vi "Main.vi"() -> ()   [LabVIEW 2013]
panel:
  in  "stop":bool
  out "Status:":string
  out "User Path Input":string
  out "Path":path
  in  "Notes":string
  out "Progress (At This Temp)":u8(slide) scale=0.0..100.0
  out "Progress (Total)":u8(slide) scale=0.0..100.0
  out "RTD Index":i32
  out "Relay Index":i32
  out "temp index":i32
  in  "Wirings":string[](array[string])=["2 Wire", "3 Wire"]
  in  "Loads":dbl[](array[numeric])=[0.0, 300.0]
  in  "Samples per Reading":dbl=1000.0
  in  "Soak Temps":dbl[](array[numeric])=[25.0, 35.0]
  in  "Multimeter USB Port":refnum<visa-resource-name>="USB0::0x0957::0x0607::MY47028683::INSTR"
  in  "Settling Time (s)":dbl=10.0
  in  "Relay Box COM Port":refnum<visa-resource-name>="COM4"
  in  "Relay Settings":u8[](array[numeric])=[0, 2, 8, 10] format="%08b"
  in  "Burster COM Port":refnum<visa-resource-name>="COM6"
  in  "Power Supply COM Port":refnum<visa-resource-name>="COM8"
  in  "RTD Temps":dbl[](array[numeric])=[50.0, 60.0, 70.0, 80.0, 90.0, 100.0, 110.0]
  in  "Voltages":dbl[](array[numeric])=[18.0, 24.0, 36.0]
  in  "Thermal Soak Time (m)":dbl=1.0
  in  "Thermal Chamber COM Port":refnum<visa-resource-name>="COM7"
  # "IFM TEMPERATURE SENSOR TEST PLATFORM"
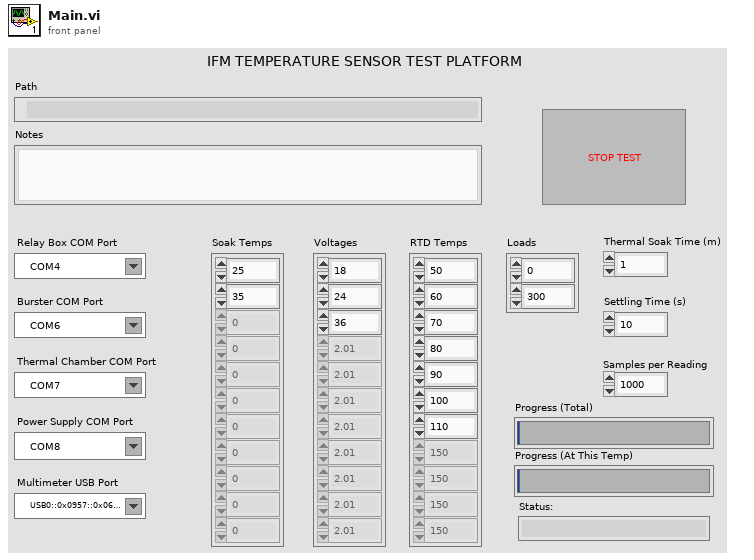
[diagram p1: front panel]
types:
  T1 = enum16{"Left Button", "Center Button", "Right Button", "Window Close"}
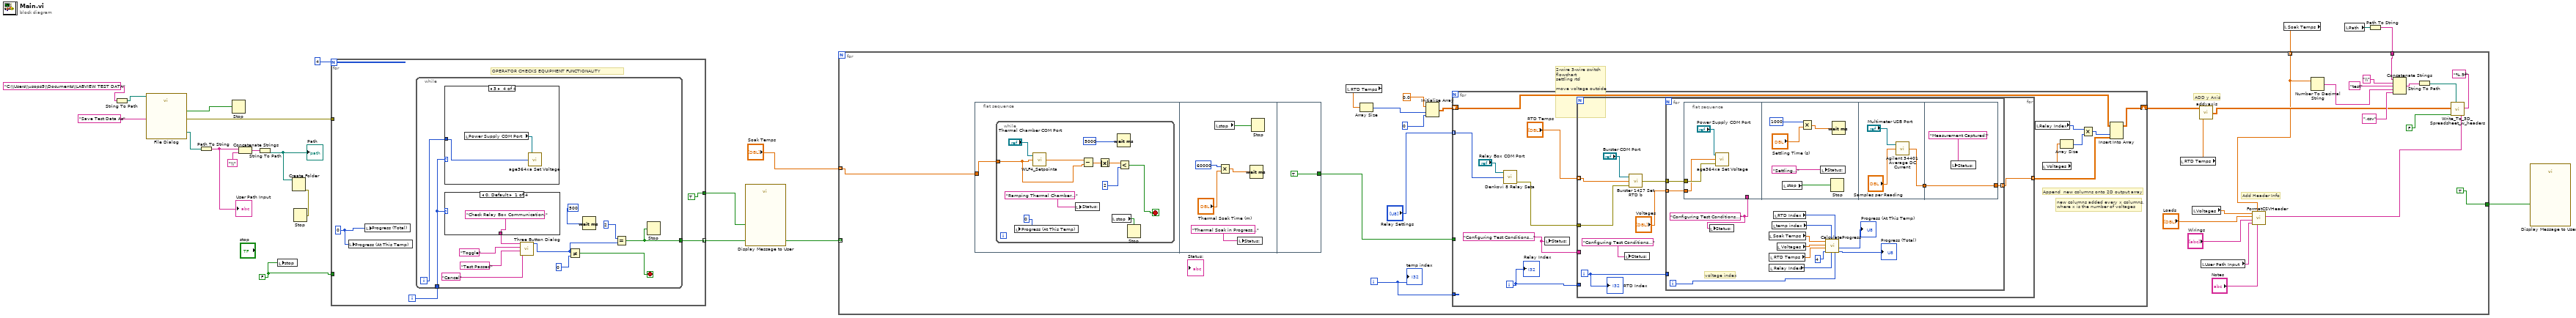
[diagram p0: block diagram]
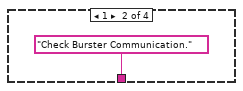
[diagram p2: hidden frame]
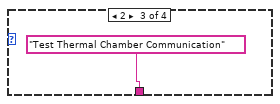
[diagram p3: hidden frame]
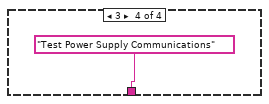
[diagram p4: hidden frame]
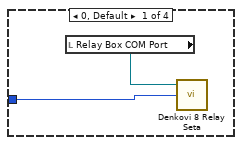
[diagram p5: hidden frame]
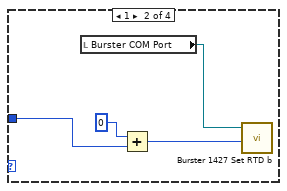
[diagram p6: hidden frame]
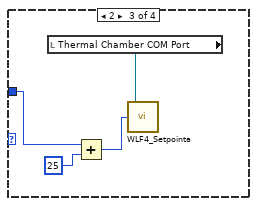
[diagram p7: hidden frame]
diagram:
  w2 = FALSE
  n1 = String To Path(string="C:\\Users\\usops5\\Documents\\LABVIEW TEST DATA") -> (path=w11:path)
  n2 = call "File Dialog"("start path"=w11, "prompt"="Save Test Data As") -> ("selected path"=w13:path, "cancelled"=w14:bool, "error out"=w15:errorcluster)  [unwired: 10 in, 1 out]
  n3 = Path To String(path=w13) -> (string=w4:string)
  "User Path Input" <- w4
  n4 = Stop(stop? (T)=w14) -> ()
  n5 = Concatenate Strings(w4, "\\") -> (w10:string)
  n6 = String To Path(string=w10) -> (path=w7:path)
  "Path" <- w7
  n7 = local write "stop"(w2) -> ()
  n8 = Create Folder(path (use dialog)=w7) -> (error out=w6:errorcluster)  [unwired: 2 in, 2 out]
  n9 = Stop(stop? (T)=w6) -> ()
  n10 = for {
    N: 4 -> [_]
    tunnel: [w23] -> w17 mode=indexing
    tunnel: w15 -> [_]
    tunnel: [TRUE] -> w3
    tunnel: w2 -> [_]
    i -> [w24]
    w21 = 0
    # "OPERATOR CHECKS EQUIPMENT FUNCTIONALITY"
    n11 = local write "Progress (At This Temp)"(w21) -> ()
    n12 = local write "Progress (Total)"(w21) -> ()
    n13 = while {
      tunnel: w24 -> [w26]
      tunnel: [w27] -> w23
      i -> [w30]
      stop <- w32 stop-if-true
      n14 = case shown="3" w26 {
        tunnel: w30 -> [w41 w46 w50 w52]
        frame 0, Default {
          n15 = local read "Relay Box COM Port"() -> (w42:refnum<visa-resource-name>)
          n16 = call "Denkovi 8 Relay Seta.vi"("Numeric"=w41, "VISA resource name"=w42) -> ()  [unwired: 3 in, 1 out]
        }
        frame 1 {
          n17 = local read "Burster COM Port"() -> (w43:refnum<visa-resource-name>)
          n18 = Add(x=0, y=w46) -> (x+y=w44:i32)
          n19 = call "Burster 1427 Set RTD b.vi"("RTD Setting"=w44, "VISA resource name"=w43) -> ()  [unwired: 1 in, 1 out]
        }
        frame 2 {
          n20 = local read "Thermal Chamber COM Port"() -> (w47:refnum<visa-resource-name>)
          n21 = Add(x=w50, y=25) -> (x+y=w48:i32)
          n22 = call "WLF4_Setpointa.vi"("Set Point 1"=w48, "Instrument Resource Name"=w47) -> ()  [unwired: 3 in, 1 out]
        }
        frame 3 {
          n23 = local read "Power Supply COM Port"() -> (w51:refnum<visa-resource-name>)
          n24 = call "age364xa Set Voltage.vi"("Voltage level (0.0 Volts)"=w52, "Instrument Resource Name (\"GPIB::5::INSTR\")"=w51) -> ()  [unwired: 1 in, 1 out]
        }
      }
      n25 = case shown="0, Default" w26 {
        tunnel: ["Check Relay Box Communication." "Check Burster Communication." "Test Thermal Chamber Communication" "Test Power Supply Communications"] -> w25
        frame 0, Default {
        }
        frame 1 {
        }
        frame 2 {
        }
        frame 3 {
        }
      }
      n26 = call <vilib>:"Three Button Dialog.vi"("Right Button Text (\"Cancel\")"="Cancel", "Center Button Text (\"No\")"="Test Passed", "Left Button Text (\"Yes\")"="Toggle", "message"=w25) -> ("Which Button?"=w28:T1)  [unwired: 7 in]
      n27 = Not Equal?(x=w28, y=0) -> (x != y?=w32:bool)
      n28 = Wait (ms)(milliseconds to wait=500) -> ()  [unwired: 1 out]
      n29 = Equal?(x=2, y=w28) -> (x = y?=w27:bool)
      n30 = Stop(stop? (T)=w27) -> ()
    }
  }
  n31 = call "Display Message to User"("Enable"=w3) -> ()  [unwired: 9 in, 2 out]
  n32 = local read "Soak Temps"() -> (w20:dbl[])
  n33 = local read "Path"() -> (w8:path)
  n34 = Path To String(path=w8) -> (string=w5:string)
  n35 = for {
    tunnel: "Soak Temps" -> [w81] mode=indexing
    tunnel: w5 -> [w54]
    tunnel: w20 -> [w69] mode=indexing
    tunnel: w17 -> [_] mode=indexing
    tunnel: [TRUE] -> w1
    i -> [w56]
    # "2-wire 3-wire switch\nflowchart\nsettling rtd\n\nmove voltage outside"
    # "ADD y Axis"
    # "Add Header Info"
    n36 = flat-sequence {
      tunnel: w81 -> [w82]
      tunnel: [TRUE] -> w59
      frame #0 {
        n37 = while {
          tunnel: w82 -> [w86]
          stop <- w89 stop-if-true
          n38 = local write "Progress (At This Temp)"(0) -> ()
          n39 = call "WLF4_Setpointa.vi"("Set Point 1"=w86, "Instrument Resource Name"="Thermal Chamber COM Port") -> ("Measured Temp"=w93:dbl)  [unwired: 3 in]
          n40 = local write "Status:"("Ramping Thermal Chamber...") -> ()
          n41 = Subtract(x=w93, y=w86) -> (x-y=w92:dbl)
          n42 = Absolute Value(x=w92) -> (abs(x)=w91:dbl)
          n43 = local read "stop"() -> (w83:bool)
          n44 = Wait (ms)(milliseconds to wait=5000) -> ()  [unwired: 1 out]
          n45 = Less?(x=w91, y=2) -> (x < y?=w89:bool)
          n46 = Stop(stop? (T)=w83) -> ()
        }
      }
      frame #1 {
        n47 = local read "stop"() -> (w94:bool)
        n48 = Multiply(x=60000, y="Thermal Soak Time (m)") -> (x*y=w98:dbl)
        n49 = local write "Status:"("Thermal Soak in Progress...") -> ()
        n50 = Wait (ms)(milliseconds to wait=w98) -> ()  [unwired: 1 out]
        n51 = Stop(stop? (T)=w94) -> ()
      }
      frame #2 {
      }
    }
    n52 = local read "RTD Temps"() -> (w63:dbl[])
    n53 = Array Size(array=w63) -> (size(s)=w65:i32)
    n54 = Initialize Array(0.0, w65, 0) -> (w62:dbl[][])
    n55 = for {
      tunnel: "Relay Settings" -> [w112] mode=indexing
      shift-right: [w107] -> w61
      shift-left: w62 -> [w105]
      tunnel: w59 -> [_]
      tunnel: w56 -> [_]
      i -> [w101]
      w100 = "Configuring Test Conditions..."
      # "new columns added every x columns,\nwhere x is the number of voltages"
      # "Append  new columns onto 2D output array"
      n56 = call "Denkovi 8 Relay Seta.vi"("Numeric"=w112, "VISA resource name"="Relay Box COM Port") -> ("Error Out"=w111:errorcluster)  [unwired: 3 in]
      n57 = local write "Status:"(w100) -> ()
      n58 = for {
        tunnel: w111 -> [w117]
        tunnel: [w120] -> w106 mode=indexing
        tunnel: "RTD Temps" -> [w119] mode=indexing
        tunnel: w101 -> [_]
        tunnel: w100 -> [_]
        i -> [w114]
        n59 = local write "Status:"("Configuring Test Conditions...") -> ()
        n60 = call "Burster 1427 Set RTD b.vi"("Error In"=w117, "RTD Setting"=w119, "VISA resource name"="Burster COM Port") -> ("Error Out"=w116:errorcluster)
        n61 = for {
          tunnel: [w135] -> w120 mode=indexing
          tunnel: w116 -> [w134]
          tunnel: "Voltages" -> [w133] mode=indexing
          tunnel: w114 -> [_]
          i -> [w123]
          w121 = "Configuring Test Conditions..."
          # "voltage index"
          n62 = flat-sequence {
            tunnel: w134 -> [w138]
            tunnel: w133 -> [w136]
            tunnel: w121 -> [_]
            tunnel: [w145] -> w122
            tunnel: [w148] -> w135
            tunnel: w122 -> [w148]
            frame #0 {
              n63 = call "age364xa Set Voltage.vi"("error in (no error)"=w138, "Voltage level (0.0 Volts)"=w136, "Instrument Resource Name (\"GPIB::5::INSTR\")"="Power Supply COM Port") -> ()  [unwired: 1 out]
            }
            frame #1 {
              n64 = local read "stop"() -> (w140:bool)
              n65 = Multiply(x=1000, y="Settling Time (s)") -> (x*y=w142:dbl)
              n66 = local write "Status:"("Settling...") -> ()
              n67 = Stop(stop? (T)=w140) -> ()
              n68 = Wait (ms)(milliseconds to wait=w142) -> ()  [unwired: 1 out]
            }
            frame #2 {
              n69 = call "Agilent 34401 Average DC Current.vi"("Multimeter Samples"="Samples per Reading", "VISA resource name"="Multimeter USB Port") -> ("Average"=w145:ext)  [unwired: 1 in]
            }
            frame #3 {
              n70 = local write "Status:"("Measurement Captured!") -> ()
            }
          }
          n71 = local write "Status:"(w121) -> ()
          n72 = local read "Soak Temps"() -> (w132:dbl[])
          n73 = local read "RTD Temps"() -> (w130:dbl[])
          n74 = local read "Relay Index"() -> (w129:i32)
          n75 = local read "temp index"() -> (w128:i32)
          n76 = local read "RTD Index"() -> (w127:i32)
          n77 = local read "Voltages"() -> (w131:dbl[])
          n78 = call "CalculateProgress.vi"("Voltage Index"=w123, "RTD Index"=w127, "Relay Index"=w129, "temp index"=w128, "Relay Settings"=4, "RTD Temps"=w130, "Voltages"=w131, "Soak Temps"=w132) -> ("Percent of Total"=→"Progress (Total)":u8, "Percent at Given Temp"=→"Progress (At This Temp)":u8)  [unwired: 2 out]
        }
        "RTD Index" <- w114
      }
      n79 = local read "Relay Index"() -> (w102:i32)
      n80 = local read "Voltages"() -> (w109:dbl[])
      n81 = Array Size(array=w109) -> (size(s)=w108:i32)
      n82 = Multiply(x=w102, y=w108) -> (x*y=w104:i32)
      n83 = Insert Into Array(array=w105, index (col)=w104, new element=w106) -> (w107:dbl[][])  [unwired: 1 in]
      "Relay Index" <- w101
    }
    n84 = local read "RTD Temps"() -> (w60:dbl[])
    n85 = local read "Voltages"() -> (w72:dbl[])
    n86 = call "addyaxis.vi"("y axis labels"=w60, "input array"=w61) -> ("Array"=w74:dbl[][])  [unwired: 1 in]
    n87 = local read "User Path Input"() -> (w57:string)
    n88 = call "FormatCSVHeader.vi"("Notes"="Notes", "Temp"=w69, "Test Path"=w57, "Wirings"="Wirings", "Loads"="Loads", "Voltages"=w72) -> ("Output String"=w68:string)  [unwired: 5 in]
    n89 = Number To Decimal String(number=w69) -> (decimal integer string=w75:string)  [unwired: 1 in]
    n90 = Concatenate Strings(w54, "\\", "test", w75, ".csv") -> (w80:string)
    n91 = String To Path(string=w80) -> (path=w77:path)
    n92 = call "Write_To_3D_Spreadsheet_w_headers.vi"("Header1"=w68, "format (%.3f)"="%.9f", 4:w77, "append to file? (new file:F)"=FALSE, "2D data"=w74) -> ()  [unwired: 3 in, 1 out]
    "temp index" <- w56
  }
  n93 = call "Display Message to User2"("Enable"=w1) -> ()  [unwired: 9 in, 2 out]
